vi "RedPrograme.vi"(8 "error in (no error)":errorcluster caption="错误输入（无错误）", 10 "字符串":string, 11 "组合框":string(combo)="R_PATH") -> (0 "error out":errorcluster caption="错误输出", 1 "filename without extension":string caption="无扩展名的文件名", 2 "value":string caption="值", 3 "file or folder exists?":bool caption="文件或文件夹存在？")   [LabVIEW 2018]
uses:
  <vilib>/Utility/config.llb/Write Key (String).vi
  <vilib>/Utility/config.llb/Read Key (String).vi
  <vilib>/Utility/config.llb/NI_LVConfig.lvlib
panel:
  out "x != y?":bool
  out "file or folder exists? 2":bool caption="文件或文件夹存在？"
  out "添加的路径":path
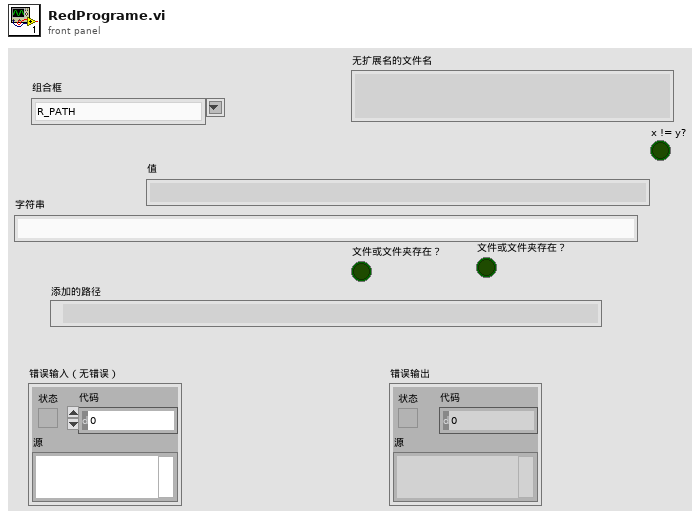
[diagram p1: front panel]
types:
  T1 = typedef "NI_LVConfig.lvlib/Config Data RefNum.ctl" = refnum<k1>
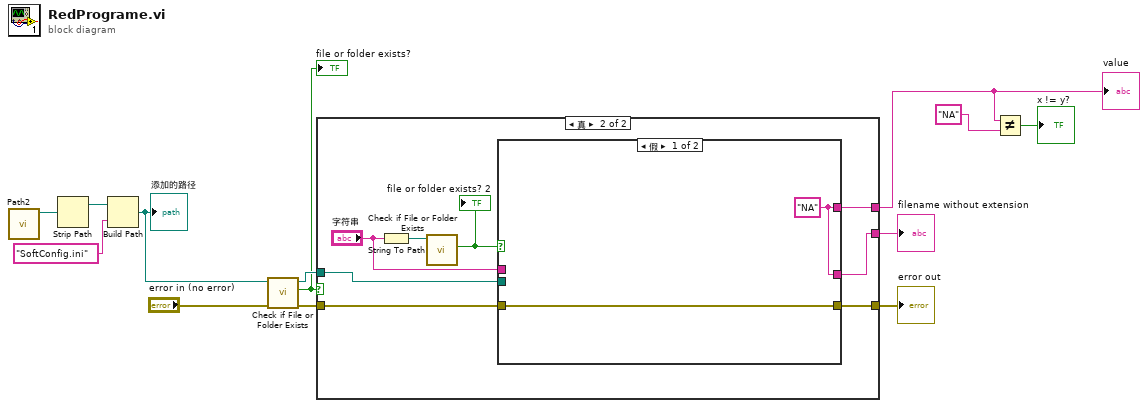
[diagram p0: block diagram]
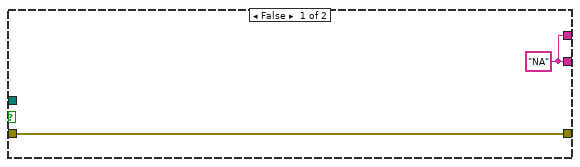
[diagram p2: hidden frame]
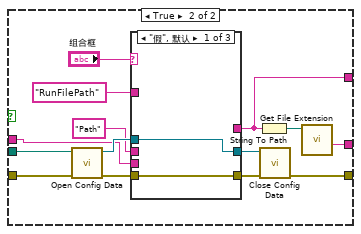
[diagram p3: hidden frame]
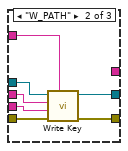
[diagram p4: hidden frame]
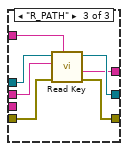
[diagram p5: hidden frame]
diagram:
  n1 = call "Path2.vi"() -> ("拆分的路径"=w11:path)  [unwired: 10 in, 1 out]
  n2 = Strip Path(path=w11) -> (stripped path=w12:path)  [unwired: 1 out]
  n3 = Build Path(base path=w12, name or relative path="SoftConfig.ini" ("名称或相对路径")) -> (appended path=w9:path)
  "添加的路径" <- w9
  n4 = call <vilib>:"Check if File or Folder Exists.vi"("error in (no error)"="error in (no error)", "path"=w9) -> ("error out"=w7:errorcluster, "file or folder exists?"=w6:bool, "dup path"=w10:path)  [unwired: 7 in]
  "file or folder exists?" <- w6
  n5 = case shown="真" w6 {
    tunnel: w7 -> [w15 w23]
    tunnel: [w15 w22] -> w5
    tunnel: w10 -> [_ w21]
    tunnel: [w14 w20] -> w4
    tunnel: [w14 w19] -> w3
    frame False {
      w14 = "NA" ("filename without extension")
    }
    frame True {
      n6 = String To Path(string="字符串") -> (path=w17:path)
      n7 = call <vilib>:"Check if File or Folder Exists.vi"("path"=w17) -> ("file or folder exists?"=w16:bool)  [unwired: 8 in, 2 out]
      "file or folder exists? 2" <- w16
      n8 = case shown="假" w16 {
        tunnel: w23 -> [w24 w32]
        tunnel: [w24 w31] -> w22
        tunnel: w21 -> [_ w30]
        tunnel: [w25 w29] -> w20
        tunnel: [w25 w27] -> w19
        tunnel: "字符串" -> [_ w26]
        frame False {
          w25 = "NA" ("filename without extension")
        }
        frame True {
          n9 = call <vilib>:"Open Config Data.vi"("error in (no error)"=w32, "configuration file path"=w30) -> ("error out"=w34:errorcluster, "refnum"=w39:T1)  [unwired: 7 in, 1 out]
          n10 = case shown="\"假\", 默认" "组合框" {
            tunnel: w39 -> [w40 w47 w55]
            tunnel: [w40 w46 w54] -> w38
            tunnel: "RunFilePath" ("section") -> [_ w45 w53]
            tunnel: "Path" ("key") -> [_ w48 w52]
            tunnel: w34 -> [w41 w44 w51]
            tunnel: [w41 w43 w50] -> w33
            tunnel: w26 -> [_ w42 _]
            tunnel: [_ _ w49] -> w27
            frame "假", Default {
            }
            frame "W_PATH" {
              n11 = call-poly <vilib>:"Write Key.vi"("section"=w45, "error in (no error)"=w44, "value"=w42, "key"=w48, "refnum"=w47) -> ("error out"=w43:errorcluster, "refnum out"=w46:T1)  [unwired: 4 in, 1 out]
            }
            frame "R_PATH" {
              n12 = call-poly <vilib>:"Read Key.vi"("section"=w53, "error in (no error)"=w51, "key"=w52, "refnum"=w55) -> ("error out"=w50:errorcluster, "value"=w49:string, "refnum out"=w54:T1)  [unwired: 4 in, 1 out]
            }
          }
          n13 = String To Path(string=w27) -> (path=w28:path)
          n14 = call <vilib>:"Close Config Data.vi"("error in (no error)"=w33, "refnum"=w38) -> ("error out"=w31:errorcluster)  [unwired: 8 in, 1 out]
          n15 = call <vilib>:"Get File Extension.vi"("file"=w28) -> ("filename without extension"=w29:string)  [unwired: 6 in, 4 out]
        }
      }
    }
  }
  "error out" <- w5
  "filename without extension" <- w4
  "value" <- w3
  n16 = Not Equal?(x=w3, y="NA" ("filename without extension")) -> (x != y?=→"x != y?":bool)
